vi "Initialization VI.vi"(8 "error in (no error)":errorcluster, 10 "Custom XML":string, 11 "Device Item Ref in":T1 format="%.0x") -> (0 "error out":errorcluster, 3 "Device Item Ref out":T1 format="%.0x")   [LabVIEW 2015, in "Inline Async Example System Explorer.lvlib"]
uses:
  Inline Async Example System Explorer.lvlib
  <vilib>/NI Veristand/Custom Device API/Custom Device Item Ref.ctl
  <vilib>/NI Veristand/Custom Device API/Custom Device Channel.ctl
  <vilib>/NI Veristand/Custom Device API/Custom Device Channel Type.ctl
  <vilib>/NI Veristand/Custom Device API/Custom Device API.lvlib
  <vilib>/NI Veristand/Custom Device Tools/Custom Device Utility Library/Custom Device Utility Library.lvlib
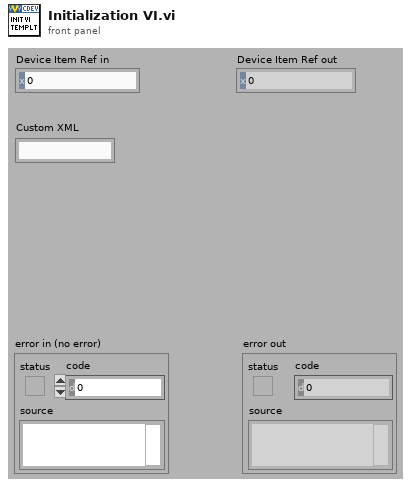
[diagram p1: front panel]
types:
  T1 = typedef "Custom Device API.lvlib/Custom Device Item Ref.ctl" = u64
  T2 = typedef "Custom Device API.lvlib/Custom Device Channel.ctl" = cluster{"Type":T3, "Units":string, "Default Value":dbl, "Faultable":bool, "Scalable":bool}
  T3 = typedef "Custom Device API.lvlib/Custom Device Channel Type.ctl" = enum16{"Input", "Output"}
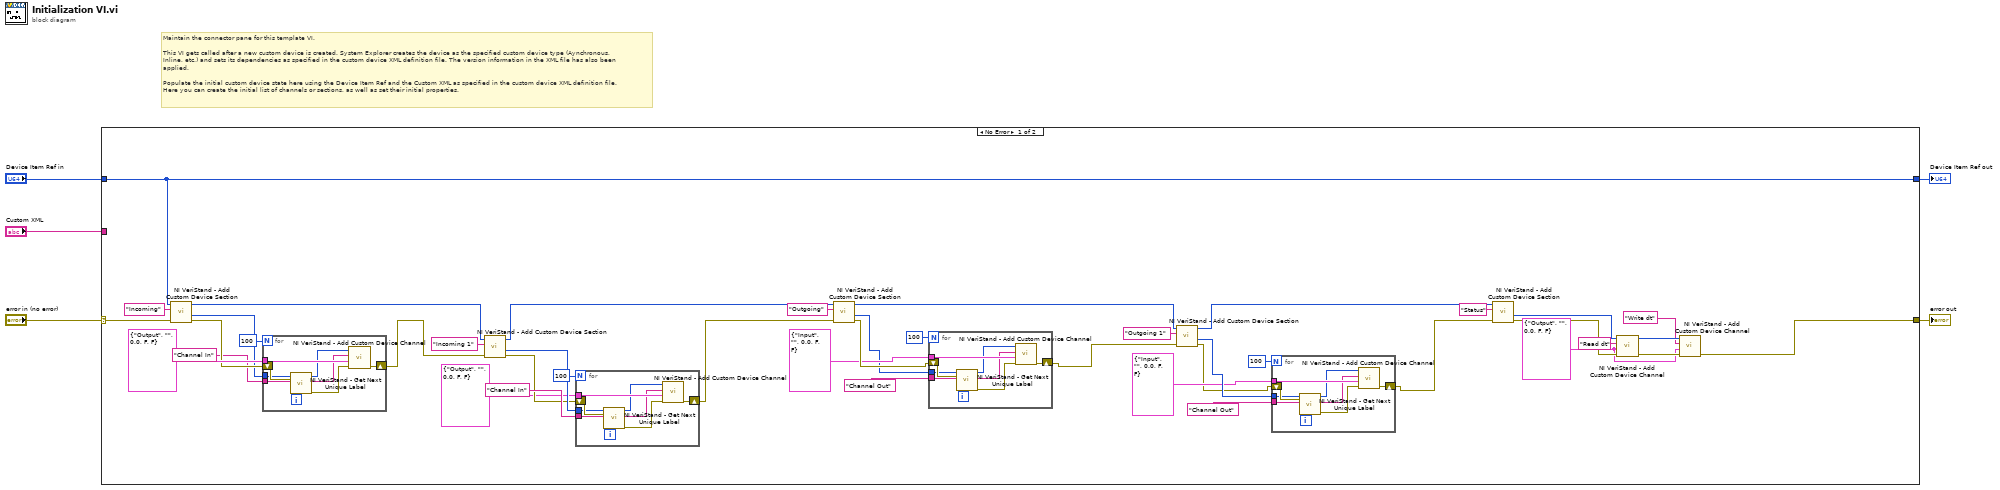
[diagram p0: block diagram]
diagram:
  # "Maintain the connector pane for this template VI.\n\nThis VI gets called after a new custom device is created. System Explorer creates the device as the specified custom device type (Aynchronous, Inline, etc.) and sets its dependencies as specified in the custom device XML definition file. The version information in the XML file has also been applied.\n\nPopulate the initial custom device state here using the Device Item Ref and the Custom XML as specified in the custom device XML definition file. Here you can create the initial list of channels or sections, as well as set their initial properties."
  n1 = case shown="No Error" "error in (no error)" {
    selector: "error in (no error)" -> [w48 w82]
    tunnel: [w37 w82] -> w5
    tunnel: [w47 w81] -> w3
    tunnel: "Device Item Ref in" -> [w47 w81]
    tunnel: "Custom XML" -> [_ _]
    frame No Error {
      w35 = T2 {"Type"=enum."Output", "Units"="", "Default Value"=0.0, "Faultable"=FALSE, "Scalable"=FALSE} ("Channel")
      n2 = call <vilib>:"NI VeriStand - Add Custom Device Section.vi"("error in (no error)"=w48, "Section Name"="Incoming", "Parent Ref in"=w47) -> ("error out"=w34:errorcluster, "Section Ptr"=w33:T1, "Parent Ref out"=w17:T1)  [unwired: 5 in, 1 out]
      n3 = for {
        N: 100 -> [_]
        tunnel: T2 {"Type"=enum."Output", "Units"="", "Default Value"=0.0, "Faultable"=FALSE, "Scalable"=FALSE} ("Channel") -> [w80]
        tunnel: w33 -> [w76]
        tunnel: "Channel In" ("Channel Name") -> [w74]
        shift-right: [w79] -> w19
        shift-left: w34 -> [w78]
        n4 = call <vilib>:"NI VeriStand - Get Next Unique Label.vi"("error in (no error)"=w78, "Label"=w74, "Parent Ref in"=w76) -> ("error out"=w77:errorcluster, "Label out"=w73:string, "Parent Ref dup"=w75:T1)  [unwired: 5 in, 1 out]
        n5 = call <vilib>:"NI VeriStand - Add Custom Device Channel.vi"("error in (no error)"=w77, "Channel"=w80, "Channel Name"=w73, "Parent Ref in"=w75) -> ("error out"=w79:errorcluster)  [unwired: 4 in, 3 out]
      }
      n6 = call <vilib>:"NI VeriStand - Add Custom Device Section.vi"("error in (no error)"=w19, "Section Name"="Incoming 1", "Parent Ref in"=w17) -> ("error out"=w22:errorcluster, "Section Ptr"=w23:T1, "Parent Ref out"=w16:T1)  [unwired: 5 in, 1 out]
      n7 = for {
        N: 100 -> [_]
        tunnel: T2 {"Type"=enum."Output", "Units"="", "Default Value"=0.0, "Faultable"=FALSE, "Scalable"=FALSE} ("Channel") -> [w64]
        tunnel: w23 -> [w60]
        tunnel: "Channel In" ("Channel Name") -> [w58]
        shift-right: [w63] -> w18
        shift-left: w22 -> [w62]
        n8 = call <vilib>:"NI VeriStand - Get Next Unique Label.vi"("error in (no error)"=w62, "Label"=w58, "Parent Ref in"=w60) -> ("error out"=w61:errorcluster, "Label out"=w57:string, "Parent Ref dup"=w59:T1)  [unwired: 5 in, 1 out]
        n9 = call <vilib>:"NI VeriStand - Add Custom Device Channel.vi"("error in (no error)"=w61, "Channel"=w64, "Channel Name"=w57, "Parent Ref in"=w59) -> ("error out"=w63:errorcluster)  [unwired: 4 in, 3 out]
      }
      n10 = call <vilib>:"NI VeriStand - Add Custom Device Section.vi"("error in (no error)"=w18, "Section Name"="Outgoing", "Parent Ref in"=w16) -> ("error out"=w29:errorcluster, "Section Ptr"=w26:T1, "Parent Ref out"=w9:T1)  [unwired: 5 in, 1 out]
      n11 = for {
        N: 100 -> [_]
        tunnel: T2 {"Type"=enum."Input", "Units"="", "Default Value"=0.0, "Faultable"=FALSE, "Scalable"=FALSE} ("Channel") -> [w72]
        tunnel: w26 -> [w68]
        tunnel: "Channel Out" ("Channel Name") -> [w66]
        shift-right: [w71] -> w7
        shift-left: w29 -> [w70]
        n12 = call <vilib>:"NI VeriStand - Get Next Unique Label.vi"("error in (no error)"=w70, "Label"=w66, "Parent Ref in"=w68) -> ("error out"=w69:errorcluster, "Label out"=w65:string, "Parent Ref dup"=w67:T1)  [unwired: 5 in, 1 out]
        n13 = call <vilib>:"NI VeriStand - Add Custom Device Channel.vi"("error in (no error)"=w69, "Channel"=w72, "Channel Name"=w65, "Parent Ref in"=w67) -> ("error out"=w71:errorcluster)  [unwired: 4 in, 3 out]
      }
      n14 = call <vilib>:"NI VeriStand - Add Custom Device Section.vi"("error in (no error)"=w7, "Section Name"="Outgoing 1", "Parent Ref in"=w9) -> ("error out"=w12:errorcluster, "Section Ptr"=w15:T1, "Parent Ref out"=w8:T1)  [unwired: 5 in, 1 out]
      n15 = for {
        N: 100 -> [_]
        tunnel: T2 {"Type"=enum."Input", "Units"="", "Default Value"=0.0, "Faultable"=FALSE, "Scalable"=FALSE} ("Channel") -> [w56]
        tunnel: w15 -> [w52]
        tunnel: "Channel Out" ("Channel Name") -> [w50]
        shift-right: [w55] -> w6
        shift-left: w12 -> [w54]
        n16 = call <vilib>:"NI VeriStand - Get Next Unique Label.vi"("error in (no error)"=w54, "Label"=w50, "Parent Ref in"=w52) -> ("error out"=w53:errorcluster, "Label out"=w49:string, "Parent Ref dup"=w51:T1)  [unwired: 5 in, 1 out]
        n17 = call <vilib>:"NI VeriStand - Add Custom Device Channel.vi"("error in (no error)"=w53, "Channel"=w56, "Channel Name"=w49, "Parent Ref in"=w51) -> ("error out"=w55:errorcluster)  [unwired: 4 in, 3 out]
      }
      n18 = call <vilib>:"NI VeriStand - Add Custom Device Section.vi"("error in (no error)"=w6, "Section Name"="Status", "Parent Ref in"=w8) -> ("error out"=w41:errorcluster, "Section Ptr"=w40:T1)  [unwired: 5 in, 2 out]
      n19 = call <vilib>:"NI VeriStand - Add Custom Device Channel.vi"("error in (no error)"=w41, "Channel"=w35, "Channel Name"="Read dt", "Parent Ref in"=w40) -> ("error out"=w39:errorcluster, "Parent Ref out"=w38:T1)  [unwired: 4 in, 2 out]
      n20 = call <vilib>:"NI VeriStand - Add Custom Device Channel.vi"("error in (no error)"=w39, "Channel"=w35, "Channel Name"="Write dt", "Parent Ref in"=w38) -> ("error out"=w37:errorcluster)  [unwired: 4 in, 3 out]
    }
    frame Error {
    }
  }
  "error out" <- w5
  "Device Item Ref out" <- w3
